vi "FL_TTL_xor_with_IO_inv_config.vi"(10 "IO inversion config.":u16, 11 "TTL port(s) config to fire":u8) -> (2 "OFF config.":u32, 3 "ON config.":u32)   [LabVIEW 2018, in "Tracker.lvlib"]
uses:
  Tracker.lvlib
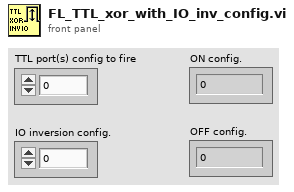
[diagram p1: front panel]
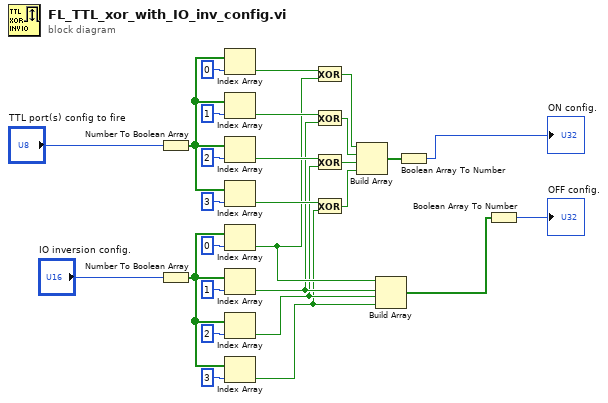
[diagram p0: block diagram]
diagram:
  n1 = Number To Boolean Array(number="TTL port(s) config to fire") -> (Boolean array=w14:bool[])
  n2 = Number To Boolean Array(number="IO inversion config.") -> (Boolean array=w12:bool[])
  n3 = Index Array(array=w14, index=0) -> (element=w7:bool)
  n4 = Index Array(array=w14, index=1) -> (element=w20:bool)
  n5 = Index Array(array=w14, index=2) -> (element=w21:bool)
  n6 = Index Array(array=w14, index=3) -> (element=w22:bool)
  n7 = Index Array(array=w12, index=0) -> (element=w5:bool)
  n8 = Index Array(array=w12, index=1) -> (element=w4:bool)
  n9 = Index Array(array=w12, index=2) -> (element=w3:bool)
  n10 = Index Array(array=w12, index=3) -> (element=w2:bool)
  n11 = Exclusive Or(1:w5, 2:w7) -> (0:w23:bool)
  n12 = Exclusive Or(1:w4, 2:w20) -> (0:w24:bool)
  n13 = Exclusive Or(1:w3, 2:w21) -> (0:w25:bool)
  n14 = Exclusive Or(1:w2, 2:w22) -> (0:w26:bool)
  n15 = Build Array(w23, w24, w25, w26) -> (w6:bool[])
  n16 = Build Array(w5, w4, w3, w2) -> (w1:bool[])
  n17 = Boolean Array To Number(Boolean array=w6) -> (number=→"ON config.":u32)
  n18 = Boolean Array To Number(Boolean array=w1) -> (number=→"OFF config.":u32)
